vi "Kill pixels +Program.vi"(0 "Layer ID list 2 (ordered)":u32[](array[numeric]) format="%.0x", 1 "All ID list 2":u32[](array[numeric]) format="%.0x", 2 "Layer ID list 1 (ordered)":u32[](array[numeric]) format="%.0x", 3 "All ID list 1":u32[](array[numeric]) format="%.0x", 4 "Addresses Cluster":T2={"ENA1"=FALSE, "IP address 1"="172.16.14.22", "ENA2"=FALSE, "IP address 2"="172.16.14.23"}, 5 "ACQ full DATA file path":path caption="File path", 7 "EQ folder path":string, 11 "Killing list A":T1(array[cluster]) {"ChipID" format="%.0x"}, 19 "Killing list B":T1(array[cluster]) {"ChipID" format="%.0x"}) -> ()   [LabVIEW 2015, in "VIPM2.lvlib"]
uses:
  VIPM2.lvlib
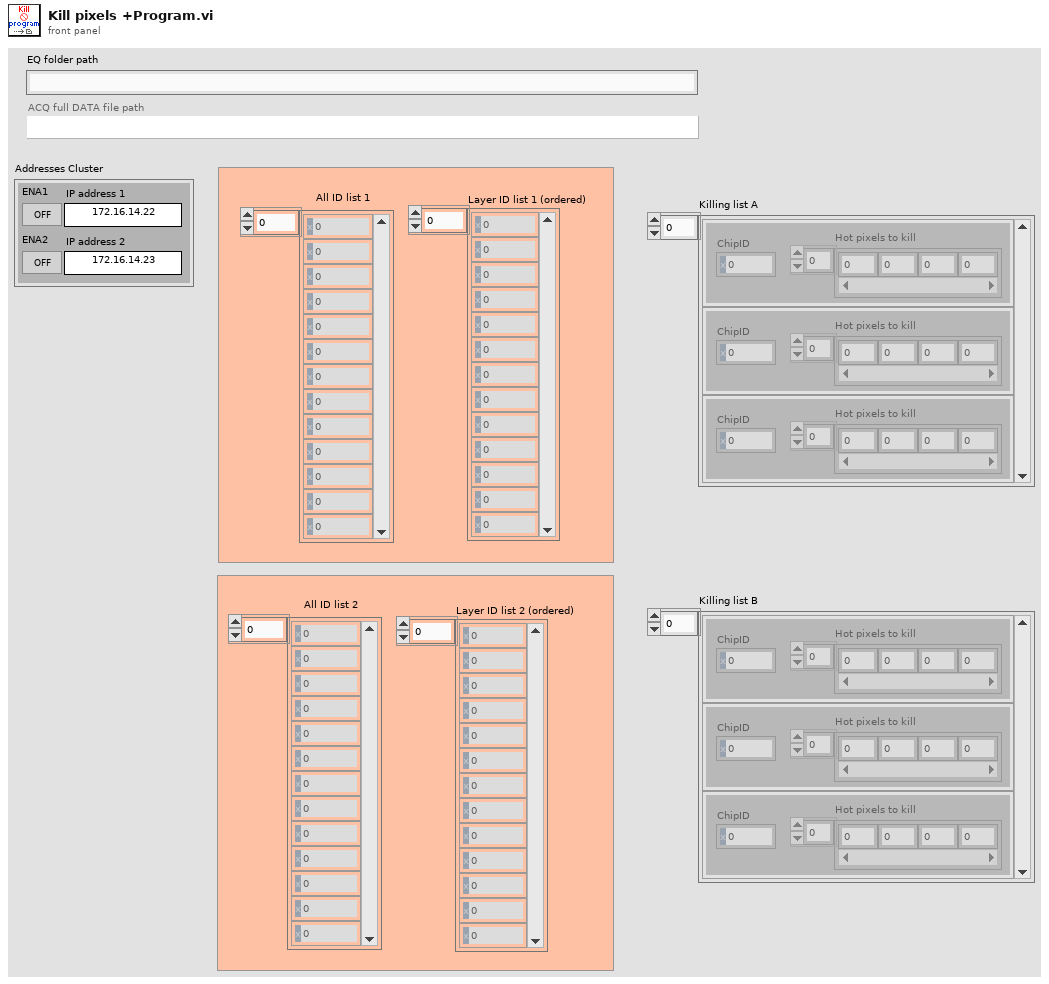
[diagram p1: front panel]
types:
  T1 = cluster{"ChipID":u16, "Hot pixels to kill":u8[]}[]
  T2 = cluster{"ENA1":bool, "IP address 1":string, "ENA2":bool, "IP address 2":string}
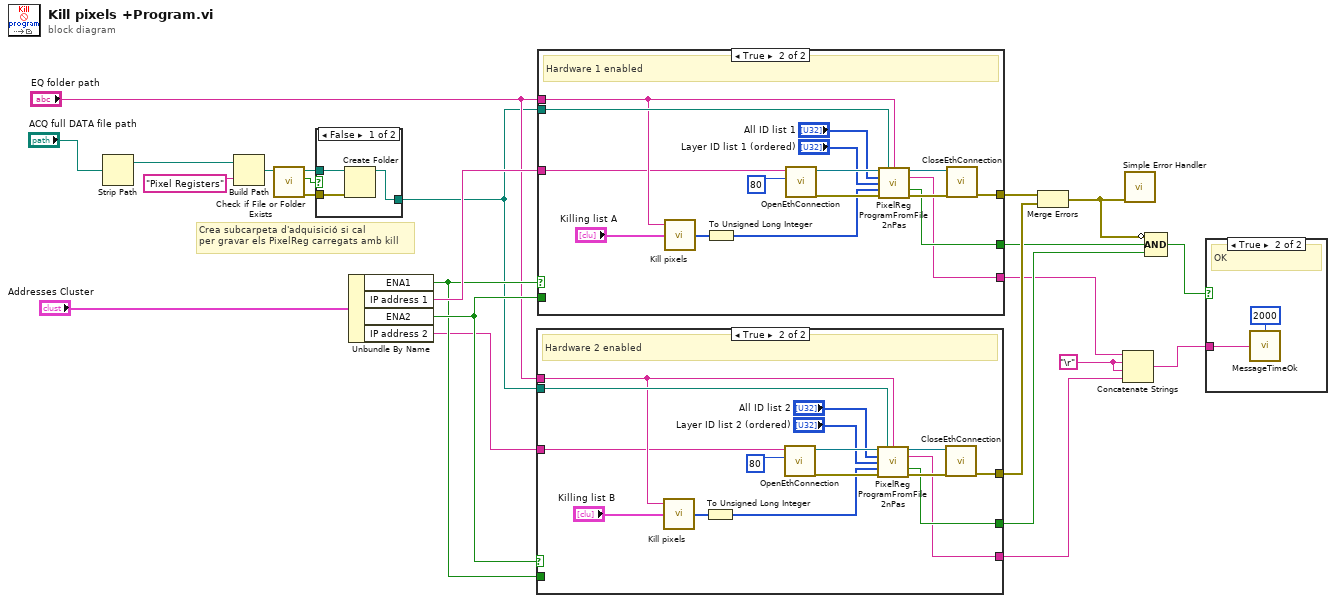
[diagram p0: block diagram]
diagram:
  w17 = "\r"
  # "Crea subcarpeta d'adquisició si cal\nper gravar els PixelReg carregats amb kill"
  n1 = Strip Path(path="ACQ full DATA file path") -> (stripped path=w2:path)  [unwired: 1 out]
  n2 = Build Path(base path=w2, name or relative path="Pixel Registers") -> (appended path=w7:path)
  n3 = call <vilib>:"Check if File or Folder Exists.vi"("path"=w7) -> ("error out"=w4:errorcluster, "file or folder exists?"=w6:bool, "dup path"=w5:path)  [unwired: 8 in]
  n4 = case shown="False" w6 {
    tunnel: w5 -> [w27 w28]
    tunnel: w4 -> [w26 _]
    tunnel: [w25 w28] -> w1
    frame False {
      n5 = Create Folder(path (use dialog)=w27, error in=w26) -> (created path=w25:path)  [unwired: 1 in, 2 out]
    }
    frame True {
    }
  }
  n6 = Unbundle By Name("Addresses Cluster") -> ("ENA1"=w21:bool, "IP address 1"=w23:string, "ENA2"=w22:bool, "IP address 2"=w20:string)
  n7 = case shown="True" w22 {
    tunnel: [w29 w43] -> w11
    tunnel: [_ w42] -> w9
    tunnel: w21 -> [w29 _]
    tunnel: "EQ folder path" -> [_ w35]
    tunnel: w1 -> [_ w38]
    tunnel: w20 -> [_ w34]
    tunnel: [_ w30] -> w15
    frame False {
      # "Hardware 2 not enabled"
    }
    frame True {
      # "Hardware 2 enabled"
      n8 = call "Kill pixels.vi"("Killing list"="Killing list B", "EQ folder path"=w35) -> ("ChipIDs to reprogram"=w37:u16[])  [unwired: 3 in]
      n9 = To Unsigned Long Integer(number=w37) -> (unsigned 32bit integer=w36:u32[])
      n10 = call "OpenEthConnection.vi"("Port"=u16 80, "IP address"=w34) -> ("error out"=w40:errorcluster, "connection ID out"=w41:refnum<k5>)  [unwired: 7 in, 1 out]
      n11 = call "PixelReg ProgramFromFile 2nPas.vi"("connection ID"=w41, "ACQ PxReg folder"=w38, "EQ folder path"=w35, "All ID list"="All ID list 2", "Layer ID list"="Layer ID list 2 (ordered)", "Chip ID list"=w36, "error in (no error)"=w40) -> ("connection ID out"=w45:refnum<k5>, "done message"=w42:string, "All checks OK"=w43:bool, "error out (no error)"=w44:errorcluster)  [unwired: 4 in, 1 out]
      n12 = call "CloseEthConnection.vi"("error in (no error)"=w44, "connection ID"=w45) -> ("error out"=w30:errorcluster)  [unwired: 9 in]
    }
  }
  n13 = case shown="True" w21 {
    tunnel: [w46 w60] -> w12
    tunnel: [_ w59] -> w10
    tunnel: w22 -> [w46 _]
    tunnel: "EQ folder path" -> [_ w50]
    tunnel: w1 -> [_ w55]
    tunnel: w23 -> [_ w49]
    tunnel: [_ w47] -> w16
    frame False {
      # "Hardware 1 not enabled"
    }
    frame True {
      # "Hardware 1 enabled"
      n14 = call "Kill pixels.vi"("Killing list"="Killing list A", "EQ folder path"=w50) -> ("ChipIDs to reprogram"=w52:u16[])  [unwired: 3 in]
      n15 = To Unsigned Long Integer(number=w52) -> (unsigned 32bit integer=w51:u32[])
      n16 = call "OpenEthConnection.vi"("Port"=u16 80, "IP address"=w49) -> ("error out"=w57:errorcluster, "connection ID out"=w58:refnum<k5>)  [unwired: 7 in, 1 out]
      n17 = call "PixelReg ProgramFromFile 2nPas.vi"("connection ID"=w58, "ACQ PxReg folder"=w55, "EQ folder path"=w50, "All ID list"="All ID list 1", "Layer ID list"="Layer ID list 1 (ordered)", "Chip ID list"=w51, "error in (no error)"=w57) -> ("connection ID out"=w62:refnum<k5>, "done message"=w59:string, "All checks OK"=w60:bool, "error out (no error)"=w61:errorcluster)  [unwired: 4 in, 1 out]
      n18 = call "CloseEthConnection.vi"("error in (no error)"=w61, "connection ID"=w62) -> ("error out"=w47:errorcluster)  [unwired: 9 in]
    }
  }
  n19 = Merge Errors "Merge Errors"(w16, w15) -> (w14:errorcluster)
  n20 = Concatenate Strings "Concatenate Strings"(w10, w17, w17, w9) -> (w18:string)
  n21 = call <vilib>:"Simple Error Handler.vi"("error in (no error)"=w14) -> ()  [unwired: 4 in, 5 out]
  n22 = Compound Arithmetic op=AND(invert w14, w12, w11) -> (w13:bool)
  n23 = case shown="True" w13 {
    tunnel: w18 -> [_ w64]
    frame False {
      # "error"
    }
    frame True {
      # "OK"
      n24 = call "MessageTimeOk.vi"("time (ms)"=2000, "missage"=w64) -> ()  [unwired: 4 in]
    }
  }
